vi "Change Password Registry.vi"(11 "权限等级":u8) -> ()   [LabVIEW 2017]
panel:
  in  "取消":bool
  in  "确定":bool
  in  "再次新密码":string
  in  "新密码":string
  in  "原密码":string
  # "密码修改"
  # "请输入原密码:"
  # "请输入新密码:"
  # "请再次输入新密码:"
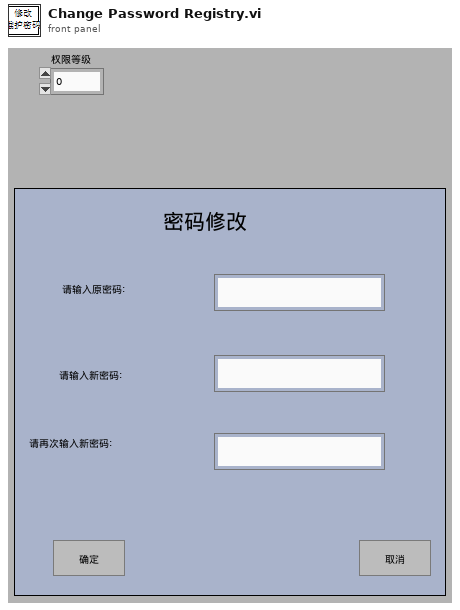
[diagram p1: front panel]
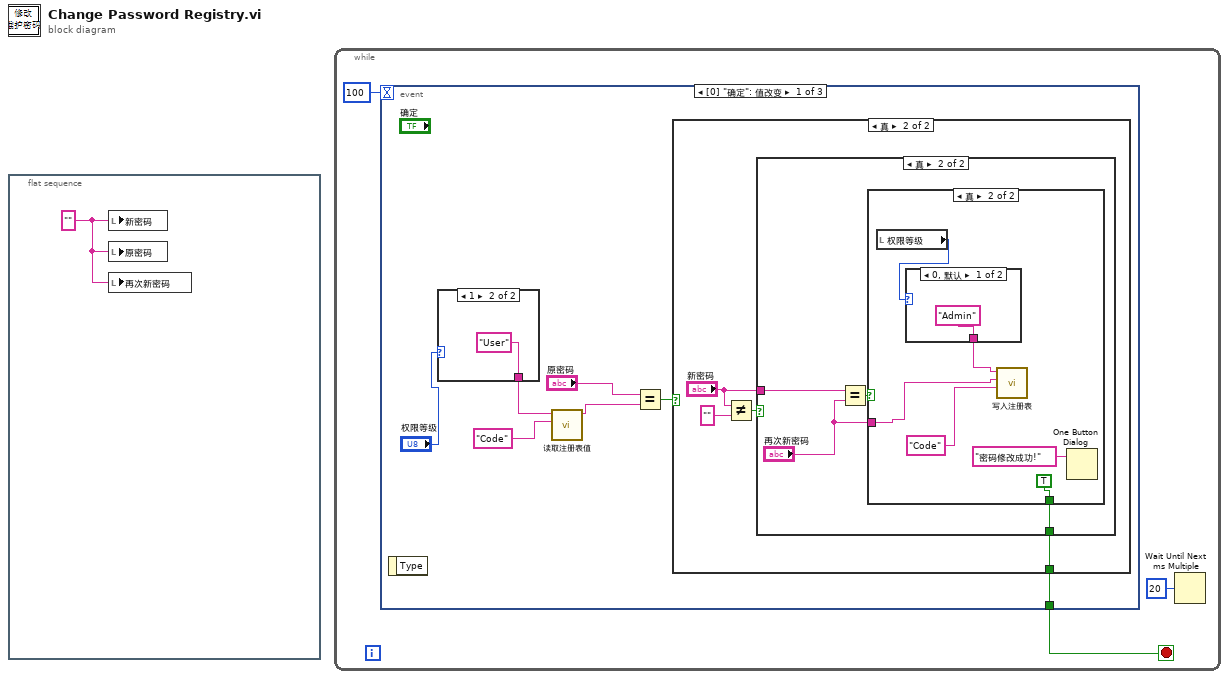
[diagram p0: block diagram]
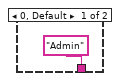
[diagram p2: hidden frame]
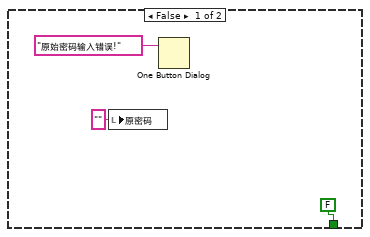
[diagram p3: hidden frame]
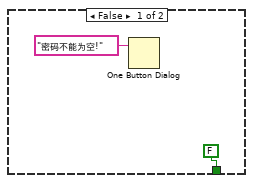
[diagram p4: hidden frame]
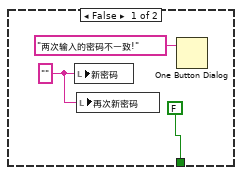
[diagram p5: hidden frame]
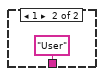
[diagram p6: hidden frame]
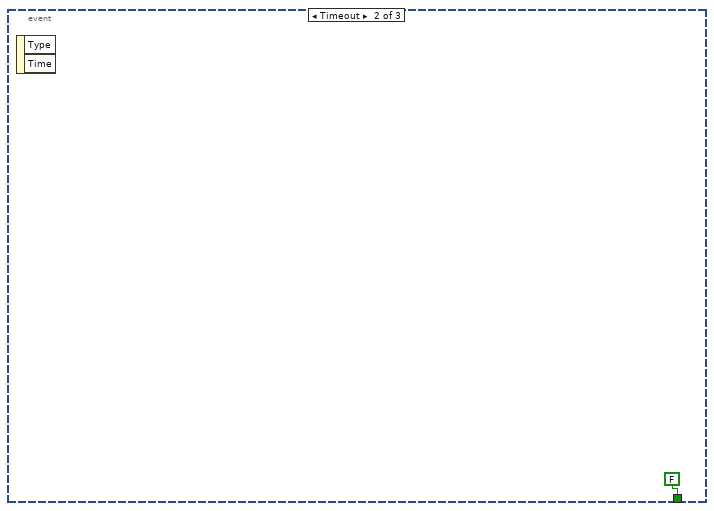
[diagram p7: hidden frame]
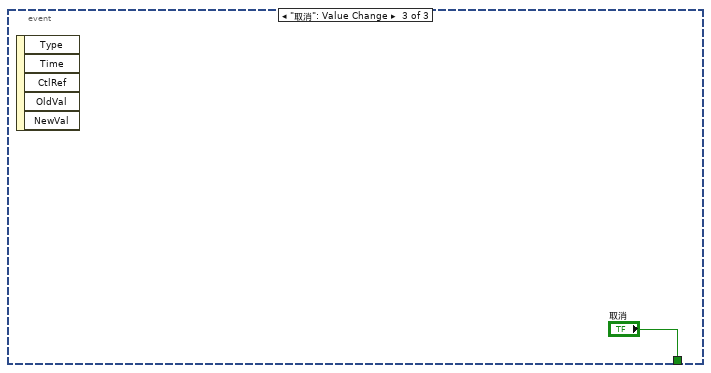
[diagram p8: hidden frame]
diagram:
  n1 = flat-sequence {
    frame #0 {
      w1 = "" ("新密码")
      n2 = local write "新密码"(w1) -> ()
      n3 = local write "原密码"(w1) -> ()
      n4 = local write "再次新密码"(w1) -> ()
    }
  }
  n5 = while {
    stop <- w4 stop-if-true
    n6 = event shown="[0] \"确定\": 值改变" {
      selector: _ -> [_ _ _]
      dyn-events: _ -> [_ _ _]
      timeout: 100 -> [_ _ _]
      tunnel: [w9 FALSE ("取消") "取消"] -> w4
      event "确定": Value Change {
        n7 = event-data() -> ()  [unwired: 1 in, 1 out]
        n8 = case shown="1" "权限等级" {
          tunnel: ["Admin" ("subkeyName") "User" ("subkeyName")] -> w6
          frame 0, Default {
          }
          frame 1 {
          }
        }
        n9 = call "读取注册表值.vi"("value"="Code", "subkeyName"=w6) -> ("Data"=w8:string)  [unwired: 7 in]
        n10 = Equal?(x="原密码", y=w8) -> (x = y?=w10:bool)
        n11 = case shown="真" w10 {
          tunnel: [FALSE ("true") w17] -> w9
          frame False {
            n12 = local write "原密码"("" ("原密码")) -> ()
            n13 = One Button Dialog(message="原始密码输入错误!") -> ()  [unwired: 1 in, 1 out]
          }
          frame True {
            n14 = Not Equal?(x="新密码", y="") -> (x != y?=w19:bool)
            n15 = case shown="真" w19 {
              tunnel: "新密码" -> [_ w26]
              tunnel: [FALSE ("true") w24] -> w17
              frame False {
                n16 = One Button Dialog(message="密码不能为空!") -> ()  [unwired: 1 in, 1 out]
              }
              frame True {
                n17 = Equal?(x=w26, y="再次新密码") -> (x = y?=w25:bool)
                n18 = case shown="真" w25 {
                  tunnel: [FALSE ("true") TRUE ("true")] -> w24
                  tunnel: "再次新密码" -> [_ w32]
                  frame False {
                    w27 = "" ("新密码")
                    n19 = local write "新密码"(w27) -> ()
                    n20 = local write "再次新密码"(w27) -> ()
                    n21 = One Button Dialog(message="两次输入的密码不一致!") -> ()  [unwired: 1 in, 1 out]
                  }
                  frame True {
                    n22 = local read "权限等级"() -> (w30:u8)
                    n23 = case shown="0, 默认" w30 {
                      tunnel: ["Admin" ("subkeyName") "User" ("subkeyName")] -> w31
                      frame 0, Default {
                      }
                      frame 1 {
                      }
                    }
                    n24 = call "写入注册表.vi"("value"="Code" ("data"), "data"=w32, "subkeyName"=w31) -> ()  [unwired: 9 in]
                    n25 = One Button Dialog(message="密码修改成功!") -> ()  [unwired: 1 in, 1 out]
                  }
                }
              }
            }
          }
        }
      }
      event Timeout {
        n26 = event-data() -> ()  [unwired: 1 in, 2 out]
      }
      event "取消": Value Change {
        n27 = event-data() -> ()  [unwired: 1 in, 5 out]
      }
    }
    n28 = Wait Until Next ms Multiple(millisecond multiple=u32 20 ("毫秒倍数")) -> ()  [unwired: 1 out]
  }
